vi "1 ch.vi"(8 "error out":errorcluster, 9 "Number of channels":i32, 11 "VISA resource name out":refnum<visa-resource-name>) -> (0 "error out 2":errorcluster, 1 "output array 3":dbl[](array[numeric]), 2 "output array 2":dbl[](array[numeric]), 3 "Means of 10":dbl[](array[numeric]), 4 "output array":dbl[](array[numeric]), 5 "VISA resource name out 2":refnum<visa-resource-name>)   [LabVIEW 2015]
uses:
  <instrlib>/Keithley 27XX/Public/Data/Read Multiple Direct.vi
  <instrlib>/Keithley 27XX/Keithley 27XX.lvlib
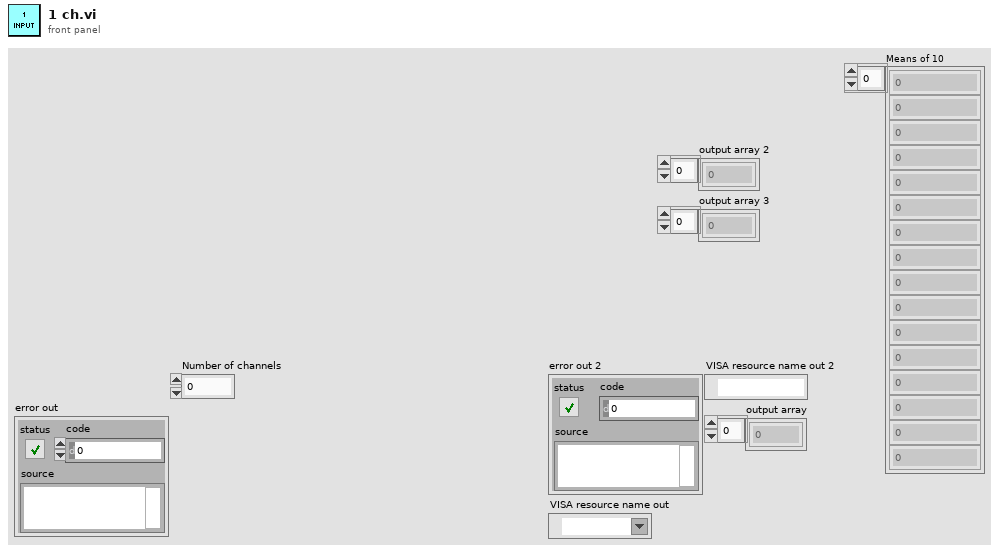
[diagram p1: front panel]
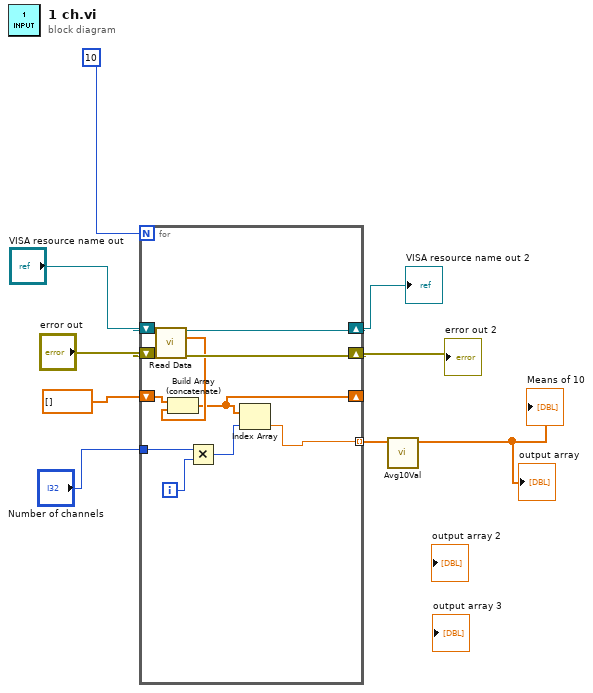
[diagram p0: block diagram]
diagram:
  n1 = for {
    N: 10 -> [_]
    shift-right: [w19] -> w8
    shift-left: "VISA resource name out" -> [w18]
    shift-right: [w20] -> w9
    shift-left: "error out" -> [w17]
    shift-right: [w11] -> _
    shift-left: dbl[] [] -> [w16]
    tunnel: "Number of channels" -> [w13]
    tunnel: [w10] -> w5 mode=indexing
    i -> [w14]
    n2 = call-poly <instrlib>:"Read Data.vi"("VISA resource name"=w18, "error in (no error)"=w17) -> ("VISA resource name out"=w19:refnum<visa-resource-name>, "Measurement Data"=w15:dbl[], "error out"=w20:errorcluster)  [unwired: 8 in, 3 out]
    n3 = Build Array (concatenate)(w16, w15) -> (w11:dbl[])
    n4 = Multiply(x=w13, y=w14) -> (x*y=w12:i32)
    n5 = Index Array(array=w11, index=w12) -> (element=w10:dbl)
  }
  "error out 2" <- w9
  "VISA resource name out 2" <- w8
  n6 = call "Avg10Val.vi"("element"=w5) -> ("Means of 10"=→"output array" →"Means of 10":dbl[])  [unwired: 10 in]
